vi "RT_R_ADC_loadcell_W_DAC.vi"() -> ()   [LabVIEW 2018]
uses:
  <vilib>/Platform/TimedLoop/XDataNode/timing_clust.ctl
  <vilib>/Platform/TimedLoop/XDataNode/nitl_modes.ctl
  <vilib>/Platform/TimedLoop/XDataNode/wakeup.ctl
  <vilib>/FPGAPlugInAG/myRIO-1900/niLvFpga_Open_myRIO-1900.vi
  <vilib>/rvi/interface/common/dynamic/niFpgaDynamicAddResources.vi
  <vilib>/Utility/error.llb/Error Cluster From Error Code.vi
  <vilib>/rvi/errors/niLvFpgaAdjustHostInterfaceError.vi
  <vilib>/FPGAPlugInAG/Dynamic/niLvFpga_Close_Dynamic.vi
  <vilib>/Platform/TimedLoop/XDataNode/XDataNode.xnode
  <vilib>/rvi/interface/nirviOpenFPGA/nirviOpenFPGA.xnode
  FPGA Bitfiles/Studentchallenge_FPGATarget_FPGARADCloadcell_UOL65CTTFtE.lvbitx
  FPGA_R_ADC_loadcell_W_DAC.vi
  <vilib>/rvi/interface/nirviReadWriteControl/nirviReadWriteControl.xnode
  <vilib>/rvi/interface/nirviCloseFPGA/nirviCloseFPGA.xnode
  <vilib>/Platform/TimedLoop/XDataNode/XDNodeRunTimeDep.lvlib
  NiFpgaLv.dll
  <vilib>/rvi/interface/Simulation/niFpgaSimulationCallBeginRW.vi
panel:
  in  "Voice coil\n input (V)":dbl
  out "Finished Late? [i-1]":bool
  out "ADC Output (V)":dbl=0.9570166470848525 format="%#.2f"
  in  "ADC Select":u16(ring)=32 items=["ADC 1"=32, "ADC 2"=40, "ADC 3"=36, "ADC 4"=44]
  in  "calibration scale":dbl=12318132.64 format="%#.6f"
  in  "calibration offset":dbl=10821562.34 format="%#.6f"
  out "Load Cell \nOutput (g)":dbl=62.20147517911448 format="%#.2f"
  in  "STOP PROGRAM":bool
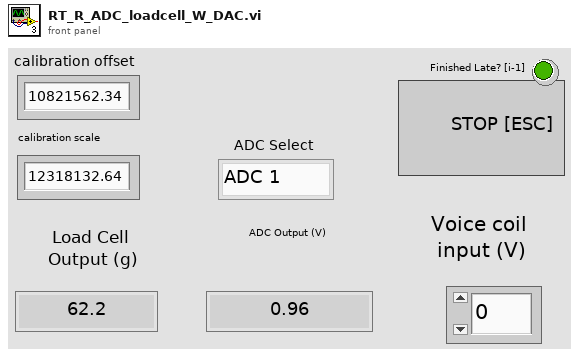
[diagram p1: front panel]
types:
  T1 = typedef "XDNodeRunTimeDep.lvlib/timing_clust.ctl" = cluster{"Expected End [f-1]":u64, "Actual End [f-1]":u64, "Finished Late? [f-1]":bool, "Expected End [i-1]":u64, "Actual End [i-1]":u64, "Finished Late? [i-1]":bool, "Expected Start [i]":u64, "Actual Start [i]":u64, "Expected Start [f]":u64, "Actual Start [f]":u64, "Source Name":string, "Structure Name":string, "Period":i64, "Deadline":i64, "Offset":i64, "Start":i64, "Priority":i32, "Timeout":i32, "Mode":T2, "Wakeup Reason":T3, "Error":errorcluster, "Source Type":string, "Secondary Source Type":string, "Global End Time":u64, "Global Start Time":u64, "Frame Duration":u64, "Iteration Duration":u64, "Assigned CPU":i32, "I/O Scan Engine Mode":u32}
  T2 = typedef "XDNodeRunTimeDep.lvlib/nitl_modes.ctl" = enum32{"No Change", "Process missed periods, maintain original phase", "Discard missed periods, maintain original phase", "Process missed periods, ignore original phase", "Discard missed periods, ignore original phase"}
  T3 = typedef "XDNodeRunTimeDep.lvlib/wakeup.ctl" = enum32{"Normal", "Aborted", "Asynchronous wakeup", "Timing source error", "Timed loop error", "Timeout"}
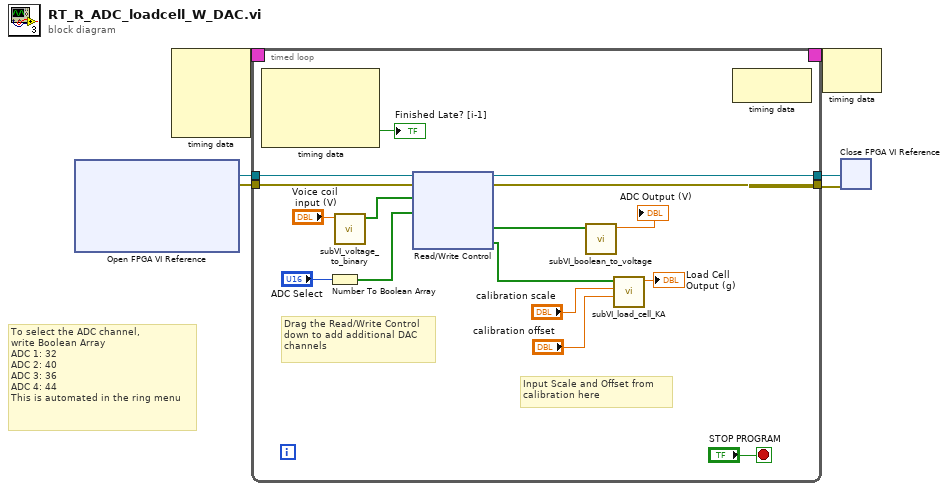
[diagram p0: block diagram]
diagram:
  # "To select the ADC channel,\nwrite Boolean Array\nADC 1: 32\nADC 2: 40\nADC 3: 36\nADC 4: 44\nThis is automated in the ring menu"
  n1 = xnode "Open FPGA VI Reference"() -> ("FPGA VI Reference Out"=w6:refnum<k20>, "error out"=w5:errorcluster)  [unwired: 2 in]
  n2 = node-c288() -> (w2:T1)  [unwired: 4 in]
  n3 = timed-loop {
    tunnel: w6 -> [w21]
    tunnel: w5 -> [w20]
    tunnel: [w17] -> w4
    tunnel: [w16] -> w3
    timing: w2 -> [_]
    timing-out: [_] -> w1
    stop <- "STOP PROGRAM" stop-if-true
    # "Input Scale and Offset from \ncalibration here"
    # "Drag the Read/Write Control\ndown to add additional DAC\nchannels"
    n4 = node-c288() -> (→"Finished Late? [i-1]":bool)  [unwired: 1 in, 3 out]
    n5 = Number To Boolean Array(number="ADC Select") -> (Boolean array=w14:bool[])
    n6 = call "subVI_voltage_to_binary.vi"("voltage"="Voice coil\n input (V)") -> ("binary"=w15:bool[])  [unwired: 10 in]
    n7 = xnode "Read/Write Control"("FPGA VI Reference In"=w21, "error in"=w20, "DAC 1 write"=w15, "ADC write"=w14) -> ("FPGA VI Reference Out"=w17:refnum<k20>, "error out"=w16:errorcluster, "ADC read"=w18:bool[], "Data array"=w13:bool[])
    n8 = call "subVI_boolean_to_voltage.vi"("ADC read"=w18) -> ("V"=→"ADC Output (V)":dbl)  [unwired: 10 in]
    n9 = call "subVI_load_cell_KA.vi"("offset"="calibration offset", "scale"="calibration scale", "DATA ARRAY IN"=w13) -> ("LOAD OUT"=→"Load Cell \nOutput (g)":dbl)  [unwired: 8 in]
    n10 = node-c288() -> ()  [unwired: 1 in, 1 out]
  }
  n11 = node-c288(w1) -> ()  [unwired: 1 out]
  n12 = xnode "Close FPGA VI Reference"("FPGA VI Reference In"=w4, "error in"=w3) -> ()  [unwired: 1 out]
